vi "Write Conversion Log File.vi"(8 "error in (no error)":errorcluster, 10 "Additional Notes?":string, 11 "Conversion.lvclass":refnum<class "Conversion.lvclass">) -> (0 "error out":errorcluster, 2 "Log File Path":path, 3 "Conversion.lvclass out":refnum<class "Conversion.lvclass">)   [LabVIEW 2016, in "Conversion.lvclass"]
uses:
  Conversion.lvclass
  Conversion.lvclass/Conversion.ctl
  <userlib>/_OpenG.lib/array/array.llb/Remove Duplicates from 1D Array (Path)__ogtk.vi
  <userlib>/_OpenG.lib/file/file.llb/Strip Path - Arrays__ogtk.vi
panel:
  in  "OK":bool
  out "resulting string":string
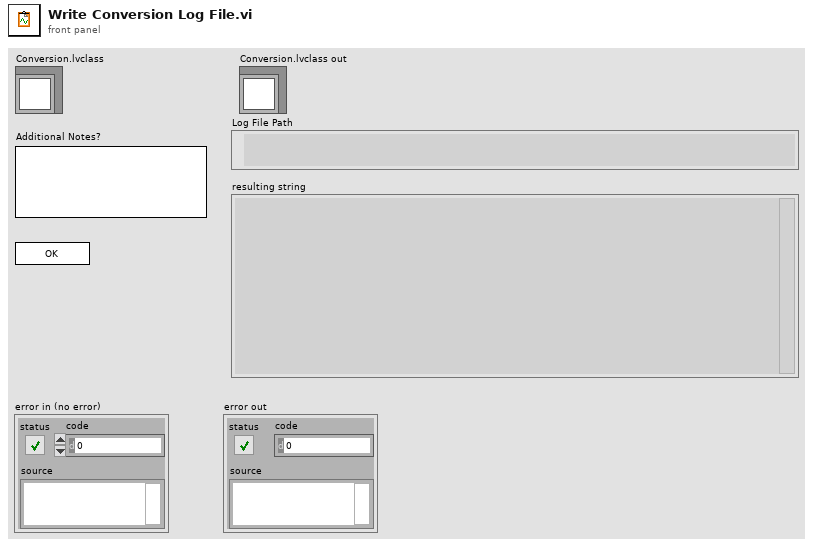
[diagram p1: front panel]
types:
  T1 = enum32{"Invalid", "Standard", "Closed", "Hidden", "Minimized", "Maximized"}
  T2 = enum32{"invalid app kind", "Development System", "Run Time System", "Student Edition", "Embedded LabVIEW", "Evaluation", "Custom"}
  T3 = cluster{"Core":cluster{"Current VI Reference":refnum<vi>, "Close Panel on Exit?":bool}, "Conversion.lvclass":refnum<class "Conversion.lvclass">, "Data.lvclass":refnum<class "Data.lvclass">, "Conversion Start time":timestamp, "Conversion End time":timestamp, "Original":path[], "Converted":path[], "Failed Conversions":path[], "Metadata":cluster{"Instrument":string, "Device":string, "Sample":string, "Experiment":string}, "Log":cluster{"Start Time":string, "End Time":string, "string":string}}
  T4 = cluster{"Instrument":string, "Device":string, "Sample":string, "Experiment":string}
  T5 = cluster{"Start Time":string, "End Time":string, "string":string}
  T6 = cluster{"Current VI Reference":refnum<vi>, "Close Panel on Exit?":bool}
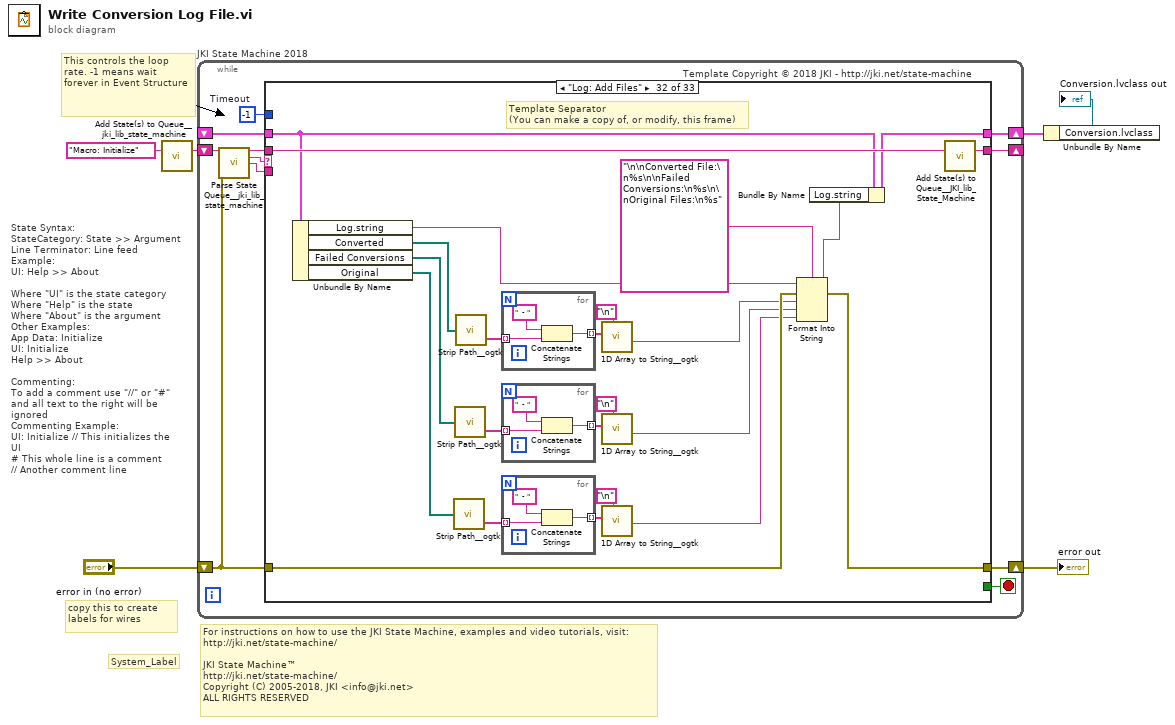
[diagram p0: block diagram]
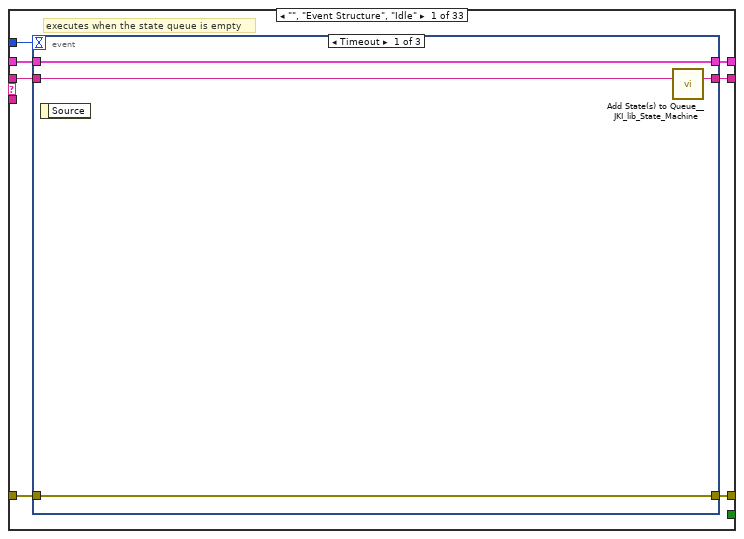
[diagram p2: hidden frame]
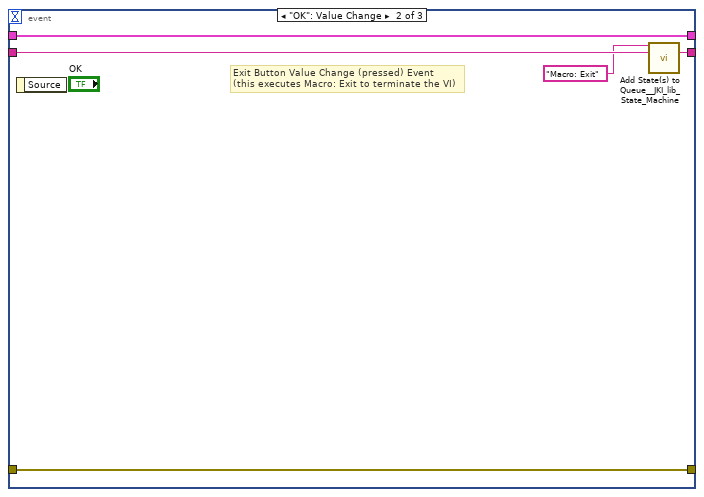
[diagram p3: hidden frame]
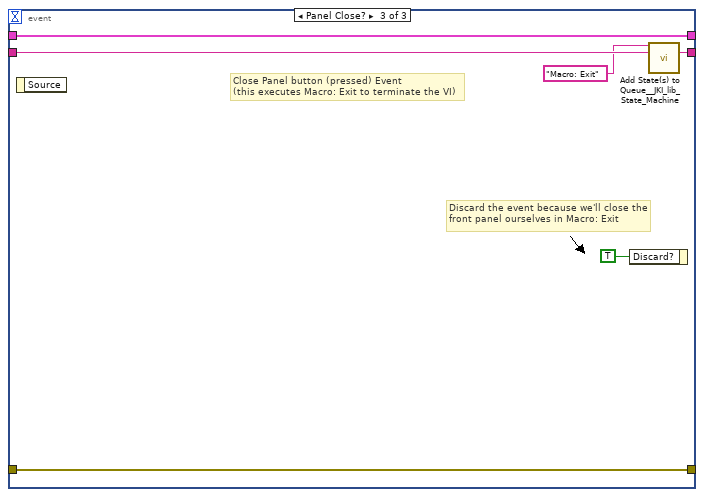
[diagram p4: hidden frame]
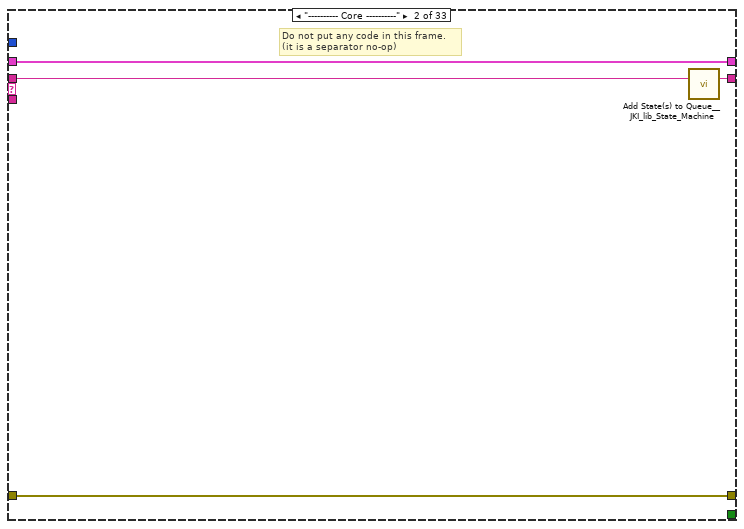
[diagram p5: hidden frame]
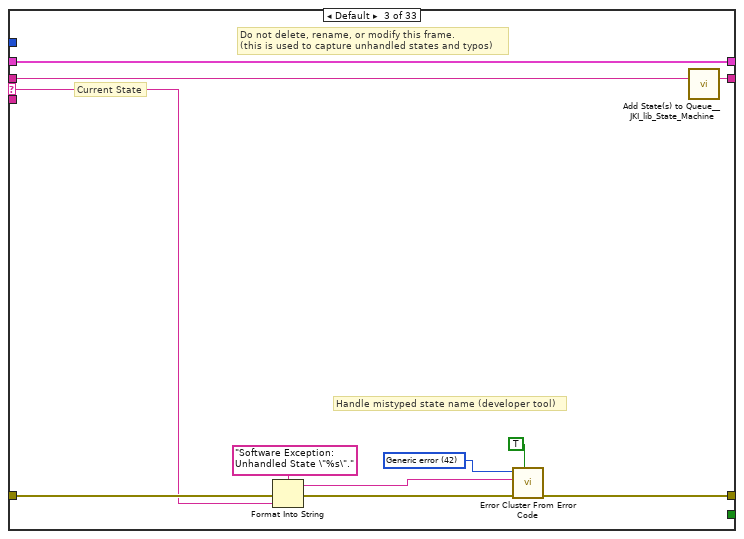
[diagram p6: hidden frame]
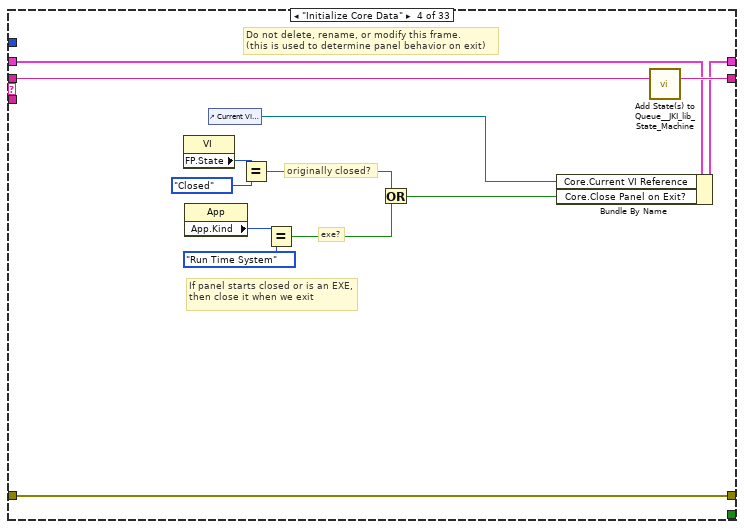
[diagram p7: hidden frame]
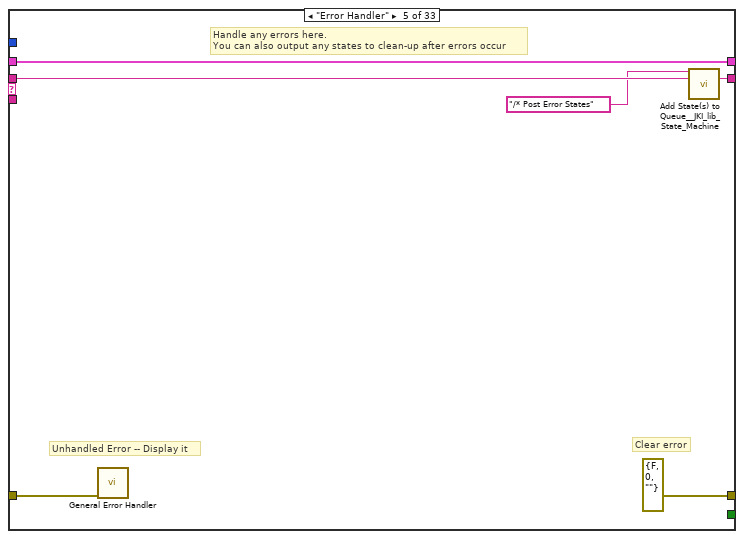
[diagram p8: hidden frame]
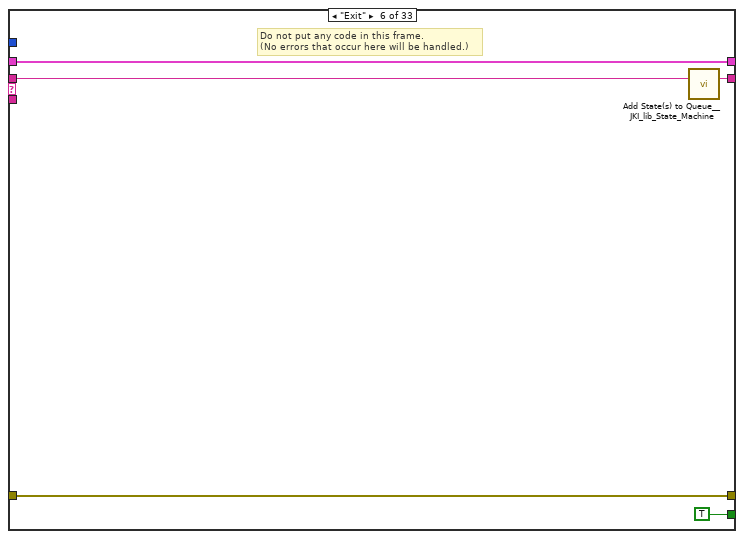
[diagram p9: hidden frame]
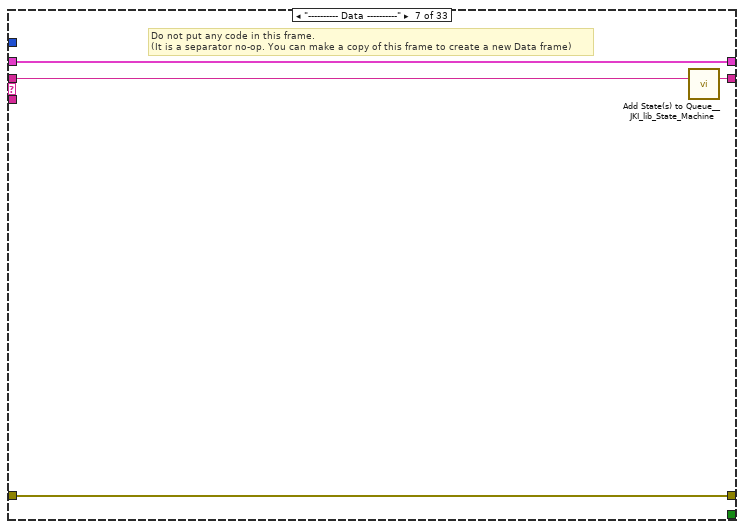
[diagram p10: hidden frame]
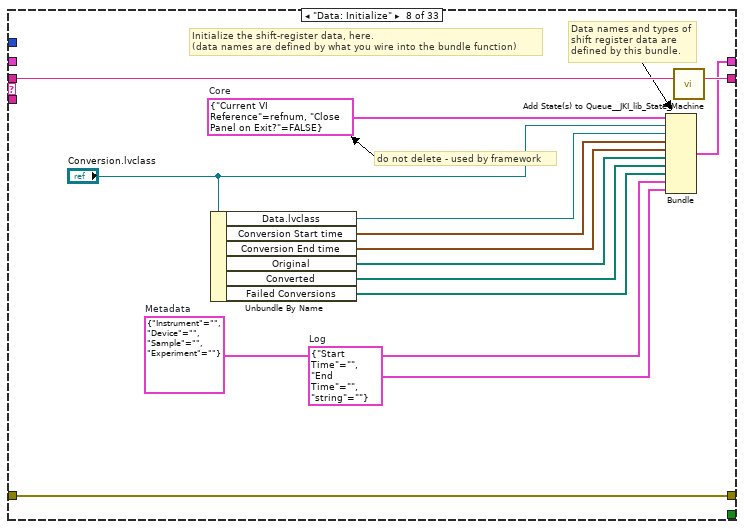
[diagram p11: hidden frame]
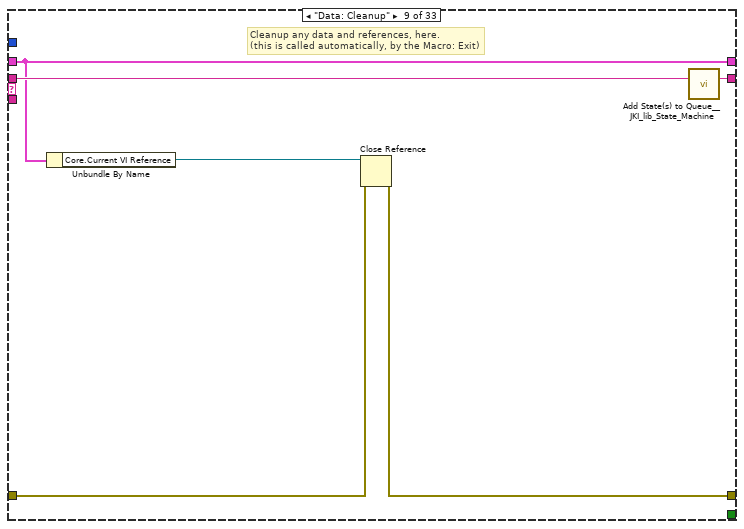
[diagram p12: hidden frame]
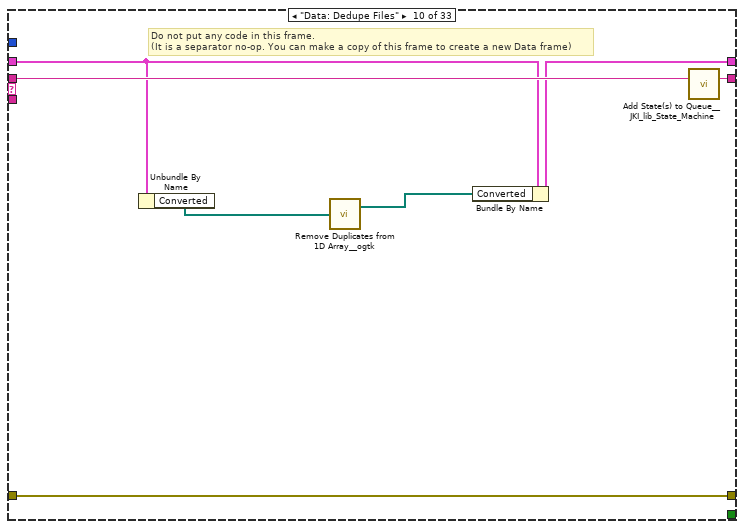
[diagram p13: hidden frame]
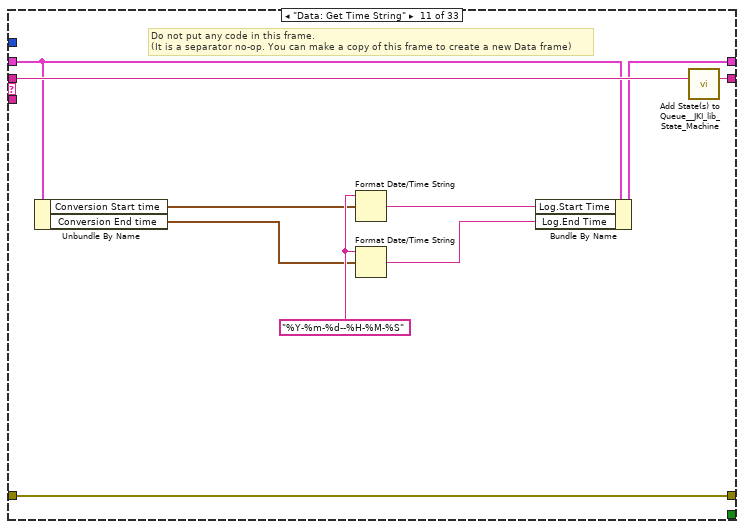
[diagram p14: hidden frame]
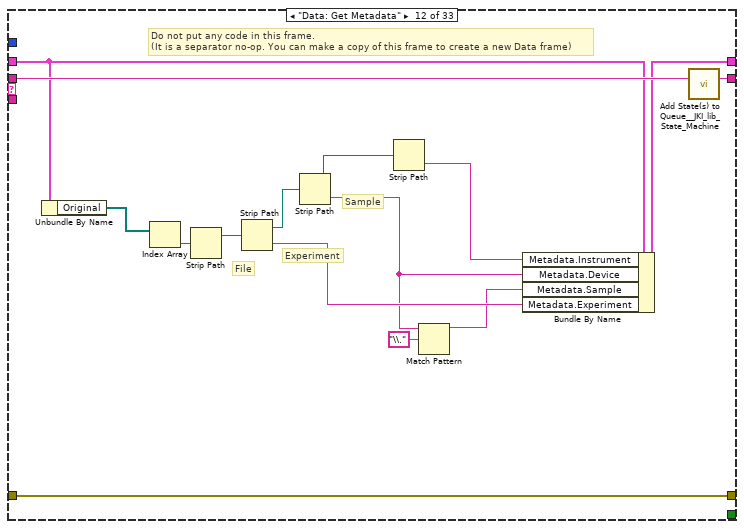
[diagram p15: hidden frame]
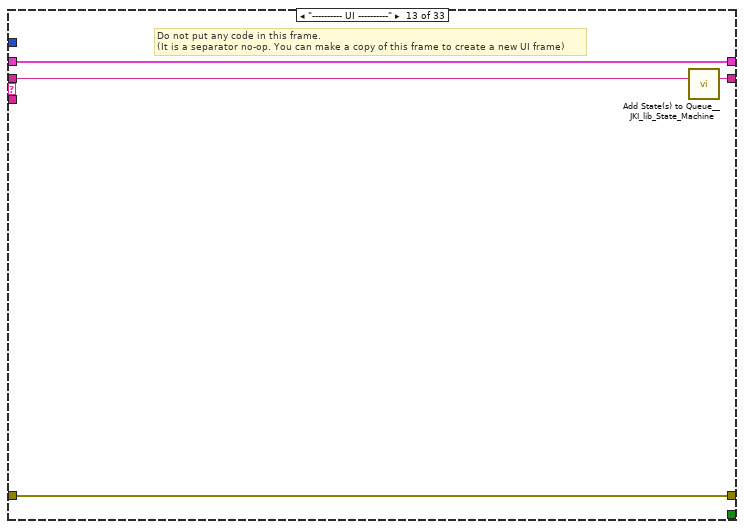
[diagram p16: hidden frame]
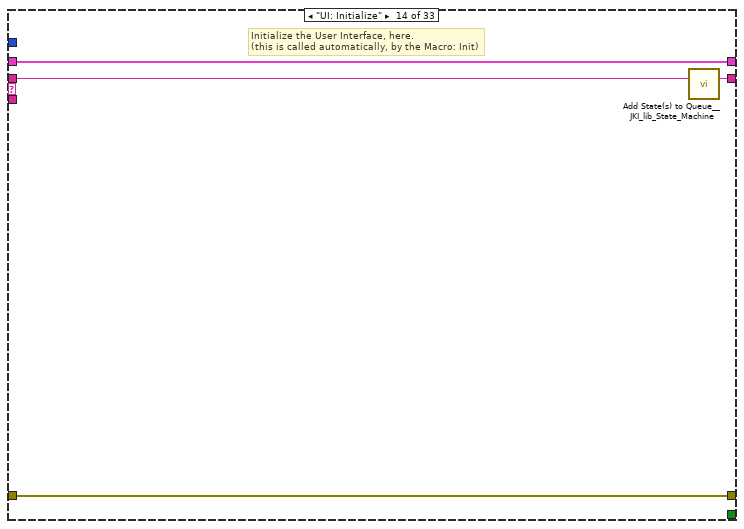
[diagram p17: hidden frame]
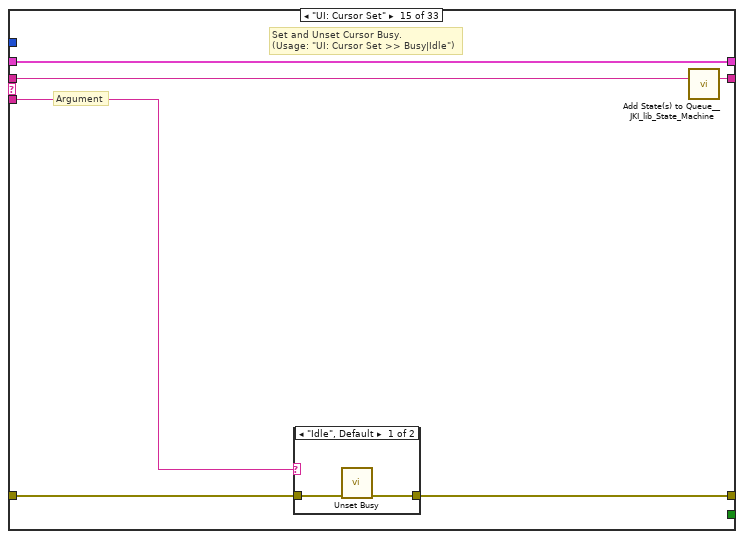
[diagram p18: hidden frame]
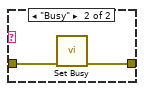
[diagram p19: hidden frame]
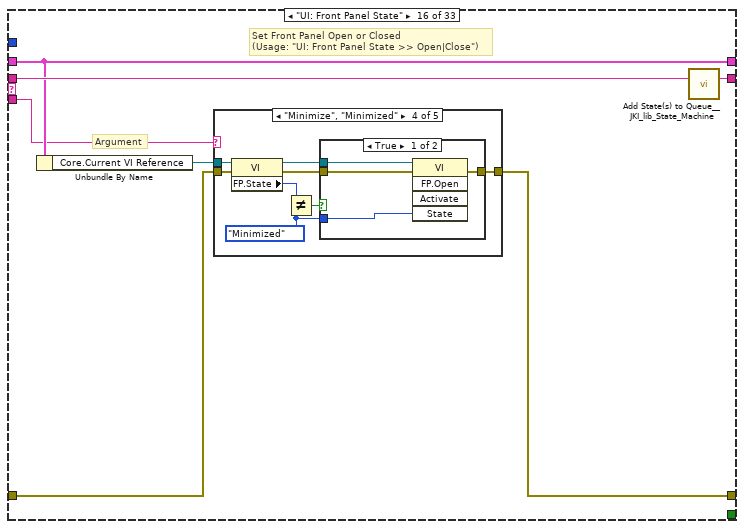
[diagram p20: hidden frame]
diagram:
  # "For instructions on how to use the JKI State Machine, examples and video tutorials, visit:\nhttp://jki.net/state-machine/\n\nJKI State Machine™\nhttp://jki.net/state-machine/\nCopyright (C) 2005-2018, JKI <info@jki.net>\nALL RIGHTS RESERVED"
  # "State Syntax:\nStateCategory: State >> Argument\nLine Terminator: Line feed\nExample:\nUI: Help >> About\n\nWhere \"UI\" is the state category\nWhere \"Help\" is the state\nWhere \"About\" is the argument\nOther Examples:\nApp Data: Initialize\nUI: Initialize\nHelp >> About\n\nCommenting:\nTo add a comment use \"//\" or \"#\" and all text to the right will be ignored\nCommenting Example:\nUI: Initialize // This initializes the UI\n# This whole line is a comment\n// Another comment line"
  # "copy this to create labels for wires"
  # "This controls the loop rate. -1 means wait forever in Event Structure"
  # "System_Label"
  n1 = call <vilib>:"Add State(s) to Queue__jki_lib_state_machine.vi"("State(s) in (\"\")"="Macro: Initialize") -> ("States Out"=w6:string)  [unwired: 14 in]
  n2 = while "JKI State Machine 2018" {
    shift-right: [w10] -> w2
    shift-left: _ -> [w9]
    shift-right: [w13] -> w4
    shift-left: "error in (no error)" -> [w7]
    shift-right: [w12] -> _
    shift-left: w6 -> [w14]
    stop <- w11 stop-if-true
    w8 = -1  # Timeout
    # "Template Copyright © 2018 JKI - http://jki.net/state-machine"
    n3 = call <vilib>:"Parse State Queue__jki_lib_state_machine.vi"("State Queue"=w14, "Error In (no error)"=w7) -> ("Remaining States"=w16:string, "Current State"=w17:string, "Arguments"=w15:string)  [unwired: 11 in]
    n4 = case shown="\"Log: Add Files\"" w17 {
      selector: w17 -> [_ _ w44 _ _ _ _ _ _ _ _ _ _ _ _ _ _ _ _ _ _ _ _ _ _ _ _ _ _ _ _ _ _]
      tunnel: w16 -> [w24 w43 w48 w67 w73 w78 w82 w96 w102 w109 w119 w134 w138 w142 w148 w159 w228 w233 w238 w248 w258 w262 w268 w278 w288 w312 w324 w335 w359 w394 w412 w447 w473]
      tunnel: w15 -> [_ _ _ _ _ _ _ _ _ _ _ _ _ _ w143 w153 _ _ _ _ _ _ _ _ _ _ _ _ _ _ _ _ _]
      tunnel: w9 -> [w22 w40 w46 w60 w70 w76 w79 _ w97 w106 w115 w126 w135 w140 w146 w155 w225 w230 w235 w245 w256 w259 w265 w276 w286 w310 w322 w333 w357 w392 w410 w445 w471]
      tunnel: [w21 w41 w50 w64 errorcluster {"status"=FALSE, "code"=0, "source"=""} ("error out") w75 w80 w93 w98 w107 w117 w132 w136 w139 w144 w156 w226 w231 w236 w246 w250 w260 w266 w271 w280 w301 w316 w327 w354 w387 w401 w440 w467] -> w13
      tunnel: w7 -> [w20 w41 w49 w64 w69 w75 w80 w93 w99 w107 w117 w132 w136 w139 w145 w157 w226 w231 w236 w246 w251 w260 w266 w272 w281 w300 w317 w328 w351 w376 w406 w441 w462]
      tunnel: [w23 w42 w47 w66 w72 w77 w81 w95 w101 w108 w118 w133 w137 w141 w147 w158 w227 w232 w237 w247 w257 w261 w267 w277 w287 w311 w323 w334 w358 w393 w411 w446 w472] -> w12
      tunnel: [_ _ _ _ _ TRUE _ _ _ _ _ _ _ _ _ _ _ _ _ _ _ _ _ _ _ _ _ _ _ _ _ _ _] -> w11
      tunnel: [w19 w40 w46 w65 w70 w76 w79 w94 w97 w104 w112 w125 w135 w140 w146 w155 w225 w230 w235 w245 w255 w259 w264 w275 w285 w309 w321 w332 w356 w391 w409 w444 w471] -> w10
      tunnel: w8 -> [w18 _ _ _ _ _ _ _ _ _ _ _ _ _ _ _ _ _ _ _ _ _ _ _ _ _ _ _ _ _ _ _ _]
      frame "", "Event Structure", "Idle" {
        # "executes when the state queue is empty"
        n5 = event shown="[0] Timeout" {
          selector: _ -> [_ _ _]
          dyn-events: _ -> [_ _ _]
          timeout: w18 -> [_ _ _]
          tunnel: w24 -> [w28 w33 w39]
          tunnel: [w27 w32 w38] -> w23
          tunnel: w22 -> [w25 w30 w36]
          tunnel: [w26 w31 w37] -> w21
          tunnel: w20 -> [w26 w31 w37]
          tunnel: [w25 w30 w36] -> w19
          event Timeout {
            n6 = event-data() -> ()  [unwired: 1 in, 1 out]
            n7 = call <vilib>:"Add State(s) to Queue__JKI_lib_State_Machine.vi"("State(s) in (\"\")"=w28) -> ("States Out"=w27:string)  [unwired: 14 in]
          }
          event "OK": Value Change {
            # "Exit Button Value Change (pressed) Event\n(this executes Macro: Exit to terminate the VI)"
            n8 = event-data() -> ()  [unwired: 1 in, 1 out]
            n9 = call <vilib>:"Add State(s) to Queue__JKI_lib_State_Machine.vi"("State(s) in Front (\"\")"="Macro: Exit", "State(s) in (\"\")"=w33) -> ("States Out"=w32:string)  [unwired: 13 in]
          }
          event Panel Close? {
            # "Discard the event because we'll close the front panel ourselves in Macro: Exit"
            # "Close Panel button (pressed) Event\n(this executes Macro: Exit to terminate the VI)"
            n10 = event-data() -> ()  [unwired: 1 in, 1 out]
            n11 = event-data("Discard?"=TRUE) -> ()  [unwired: 1 in, 1 out]
            n12 = call <vilib>:"Add State(s) to Queue__JKI_lib_State_Machine.vi"("State(s) in Front (\"\")"="Macro: Exit", "State(s) in (\"\")"=w39) -> ("States Out"=w38:string)  [unwired: 13 in]
          }
        }
      }
      frame "---------- Core ----------" {
        # "Do not put any code in this frame.\n(it is a separator no-op)"
        n13 = call <vilib>:"Add State(s) to Queue__JKI_lib_State_Machine.vi"("State(s) in (\"\")"=w43) -> ("States Out"=w42:string)  [unwired: 14 in]
      }
      frame Default {
        w53 = 42 items=["No error", "Argument error", "Memory is full", "Out of zone", "End of file", "File already open", "Generic file I/O error", "File not found", "File permission error", "Disk is full", "Duplicate path", "Too many files open", "System feature not enabled", "Resource file not found", "Cannot add resource", "Resource not found", "Image not found", "Image memory error", "Pen does not exist", "Config type invalid", "Config token not found", "Config parse error", "Config memory error", "Bad external code format", "Bad external code offset", "External code not present", "Null window", "Destroy window error", "Null menu", "Print aborted", "Bad print record", "Print driver error", "Windows error during printing", "Memory error during printing", "Print dialog error", "Generic print error", "Invalid device refnum", "Device not found", "Device parameter error", "Device unit error", "Cannot open device", "Device call aborted", "Generic error", "Cancelled by user", "Object ID too low", "Object ID too high", "Object not in heap", "Unknown heap", "Unknown object (invalid DefProc)", "Unknown object (DefProc not in table)", "Message out of range", "Invalid (null) method", "Unknown message", "Manager call not supported", "Bad address", "Network operation in progress", "Network operation timed out", "Connection is busy", "Network attribute not supported", "Network error", "Address in use", "System out of memory", "Connection aborted", "Connection refused", "Not connected", "Already connected", "Connection closed", "Initialization error (interapplication manager)", "Bad occurrence", "Wait on unbound occurrence handler", "Occurrence queue overflow", "Datalog type conflict", "Unused", "Unrecognized type (interapplication manager)", "Memory corrupt", "Failed to make temporary DLL", "Old CIN version", "Drag socket not found", "Failed to load drop-object", "Failed to register OLE object", "Failed to release OLE object", "Format specifier type mismatch", "Unknown format specifier", "Too few format specifiers", "Too many format specifiers", "Scan failed", "Newer CIN version", "Error converting to variant", "Runtime menu error", "Password tampered", "Variant attribute not found", "Incompatible variant data type", "Event data is not available", "Event Store is not present", "Occurrence is not found", "Event Queue is not created", "Event info is not available", "Refnum passed is NULL", "Error retrieving Class GUID", "Error retrieving CoClass GUID", "Error retrieving TypeLib GUID.", "Bad built application magic bytes.", "Specific driver is different from the specific driver associated with the Logical Name.", "There is no session opened to the class driver.", "Max Error", "MAX - Error with config objects", "MAX - Error loading configuration", "MAX - Group not supported"]
        # "Current State"
        # "Do not delete, rename, or modify this frame.\n(this is used to capture unhandled states and typos)"
        # "Handle mistyped state name (developer tool)"
        n14 = Format Into String(format string="Software Exception: Unhandled State \"%s\"." ("message"), error in=w49, w44) -> (resulting string=w52:string, error out=w51:errorcluster)  [unwired: 1 in]
        n15 = call <vilib>:"Error Cluster From Error Code.vi"("show call chain? (False)"=TRUE, "error in (no error)"=w51, "error message (\"\")"=w52, "error code (0)"=w53) -> ("error out"=w50:errorcluster)  [unwired: 5 in]
        n16 = call <vilib>:"Add State(s) to Queue__JKI_lib_State_Machine.vi"("State(s) in (\"\")"=w48) -> ("States Out"=w47:string)  [unwired: 14 in]
      }
      frame "Initialize Core Data" {
        # "Do not delete, rename, or modify this frame.\n(this is used to determine panel behavior on exit)"
        # "originally closed?"
        # "exe?"
        # "If panel starts closed or is an EXE, then close it when we exit"
        n17 = property class="VI"() -> ("FP.State"=w57:T1)  [unwired: 2 in, 2 out]
        n18 = property class="App"() -> ("App.Kind"=w63:T2)  [unwired: 2 in, 2 out]
        n19 = control-ref of="Current VI Reference"() -> (w58:refnum<vi>)
        n20 = Equal?(x=w57, y=T1."Closed" ("Front Panel Window:State")) -> (x = y?=w55:bool)
        n21 = Equal?(x=w63, y=T2."Run Time System" ("Application:Kind")) -> (x = y?=w61:bool)
        n22 = Or(x=w55, y=w61) -> (x .or. y?=w59:bool)
        n23 = Bundle By Name(cluster=w60, "Core.Current VI Reference"=w58, "Core.Close Panel on Exit?"=w59) -> (w65:T3)
        n24 = call <vilib>:"Add State(s) to Queue__JKI_lib_State_Machine.vi"("State(s) in (\"\")"=w67) -> ("States Out"=w66:string)  [unwired: 14 in]
      }
      frame "Error Handler" {
        # "Unhandled Error -- Display it"
        # "Handle any errors here.\nYou can also output any states to clean-up after errors occur"
        # "Clear error"
        n25 = call <vilib>:"General Error Handler.vi"("error in (no error)"=w69) -> ()  [unwired: 10 in, 5 out]
        n26 = call <vilib>:"Add State(s) to Queue__JKI_lib_State_Machine.vi"("State(s) in Front (\"\")"="/* Post Error States", "State(s) in (\"\")"=w73) -> ("States Out"=w72:string)  [unwired: 13 in]
      }
      frame "Exit" {
        # "Do not put any code in this frame.\n(No errors that occur here will be handled.)"
        n27 = call <vilib>:"Add State(s) to Queue__JKI_lib_State_Machine.vi"("State(s) in (\"\")"=w78) -> ("States Out"=w77:string)  [unwired: 14 in]
      }
      frame "---------- Data ----------" {
        # "Do not put any code in this frame.\n(It is a separator no-op. You can make a copy of this frame to create a new Data frame)"
        n28 = call <vilib>:"Add State(s) to Queue__JKI_lib_State_Machine.vi"("State(s) in (\"\")"=w82) -> ("States Out"=w81:string)  [unwired: 14 in]
      }
      frame "Data: Initialize" {
        w85 = T4 {"Instrument"="", "Device"="", "Sample"="", "Experiment"=""}  # Metadata
        w86 = T5 {"Start Time"="", "End Time"="", "string"=""}  # Log
        w92 = T6 {"Current VI Reference"=refnum, "Close Panel on Exit?"=FALSE}  # Core
        # "do not delete - used by framework"
        # "Data names and types of shift register data are defined by this bundle."
        # "Initialize the shift-register data, here.\n(data names are defined by what you wire into the bundle function)"
        n29 = Unbundle By Name("Conversion.lvclass") -> ("Data.lvclass"=w91:refnum<class "Data.lvclass">, "Conversion Start time"=w90:timestamp, "Conversion End time"=w89:timestamp, "Original"=w87:path[], "Converted"=w84:path[], "Failed Conversions"=w88:path[])
        n30 = Bundle("Core"=w92, "Conversion.lvclass"="Conversion.lvclass", "Data.lvclass"=w91, "Conversion Start time"=w90, "Conversion End time"=w89, "Original"=w87, "Converted"=w84, "Failed Conversions"=w88, "Metadata"=w85, "Log"=w86) -> (w94:T3)  [unwired: 1 in]
        n31 = call <vilib>:"Add State(s) to Queue__JKI_lib_State_Machine.vi"("State(s) in (\"\")"=w96) -> ("States Out"=w95:string)  [unwired: 14 in]
      }
      frame "Data: Cleanup" {
        # "Cleanup any data and references, here.\n(this is called automatically, by the Macro: Exit)"
        n32 = Unbundle By Name(w97) -> ("Core.Current VI Reference"=w100:refnum<vi>)
        n33 = Close Reference(reference=w100, error in (no error)=w99) -> (error out=w98:errorcluster)
        n34 = call <vilib>:"Add State(s) to Queue__JKI_lib_State_Machine.vi"("State(s) in (\"\")"=w102) -> ("States Out"=w101:string)  [unwired: 14 in]
      }
      frame "Data: Dedupe Files" {
        # "Do not put any code in this frame.\n(It is a separator no-op. You can make a copy of this frame to create a new Data frame)"
        n35 = Unbundle By Name(w106) -> ("Converted"=w105:path[])
        n36 = call-poly <userlib>:"Remove Duplicates from 1D Array__ogtk.vi"("Input Array"=w105) -> ("Output Array"=w103:path[])  [unwired: 1 out]
        n37 = Bundle By Name(cluster=w106, "Converted"=w103) -> (w104:T3)
        n38 = call <vilib>:"Add State(s) to Queue__JKI_lib_State_Machine.vi"("State(s) in (\"\")"=w109) -> ("States Out"=w108:string)  [unwired: 14 in]
      }
      frame "Data: Get Time String" {
        w116 = "%Y-%m-%d--%H-%M-%S" ("time format string (%c)")
        # "Do not put any code in this frame.\n(It is a separator no-op. You can make a copy of this frame to create a new Data frame)"
        n39 = Unbundle By Name(w115) -> ("Conversion Start time"=w114:timestamp, "Conversion End time"=w113:timestamp)
        n40 = Format Date/Time String(time format string (%c)=w116, seconds (now)=w114) -> (date/time string=w111:string)  [unwired: 1 in]
        n41 = Format Date/Time String(time format string (%c)=w116, seconds (now)=w113) -> (date/time string=w110:string)  [unwired: 1 in]
        n42 = Bundle By Name(cluster=w115, "Log.Start Time"=w111, "Log.End Time"=w110) -> (w112:T3)
        n43 = call <vilib>:"Add State(s) to Queue__JKI_lib_State_Machine.vi"("State(s) in (\"\")"=w119) -> ("States Out"=w118:string)  [unwired: 14 in]
      }
      frame "Data: Get Metadata" {
        # "Sample"
        # "Experiment"
        # "File"
        # "Do not put any code in this frame.\n(It is a separator no-op. You can make a copy of this frame to create a new Data frame)"
        n44 = Unbundle By Name(w126) -> ("Original"=w127:path[])
        n45 = Index Array(array=w127) -> (element=w130:path)  [unwired: 1 in]
        n46 = Strip Path(path=w130) -> (stripped path=w129:path)  [unwired: 1 out]
        n47 = Strip Path(path=w129) -> (stripped path=w131:path, name=w123:string)
        n48 = Strip Path(path=w131) -> (stripped path=w128:path, name=w122:string)
        n49 = Strip Path(path=w128) -> (name=w124:string)  [unwired: 1 out]
        n50 = Match Pattern(string=w122, regular expression="\\.") -> (before substring=w120:string)  [unwired: 1 in, 3 out]
        n51 = Bundle By Name(cluster=w126, "Metadata.Instrument"=w124, "Metadata.Device"=w122, "Metadata.Sample"=w120, "Metadata.Experiment"=w123) -> (w125:T3)
        n52 = call <vilib>:"Add State(s) to Queue__JKI_lib_State_Machine.vi"("State(s) in (\"\")"=w134) -> ("States Out"=w133:string)  [unwired: 14 in]
      }
      frame "---------- UI ----------" {
        # "Do not put any code in this frame.\n(It is a separator no-op. You can make a copy of this frame to create a new UI frame)"
        n53 = call <vilib>:"Add State(s) to Queue__JKI_lib_State_Machine.vi"("State(s) in (\"\")"=w138) -> ("States Out"=w137:string)  [unwired: 14 in]
      }
      frame "UI: Initialize" {
        # "Initialize the User Interface, here.\n(this is called automatically, by the Macro: Init)"
        n54 = call <vilib>:"Add State(s) to Queue__JKI_lib_State_Machine.vi"("State(s) in (\"\")"=w142) -> ("States Out"=w141:string)  [unwired: 14 in]
      }
      frame "UI: Cursor Set" {
        # "Argument"
        # "Set and Unset Cursor Busy.\n(Usage: \"UI: Cursor Set >> Busy|Idle\")"
        n55 = case shown="\"Idle\", Default" w143 {
          tunnel: w145 -> [w150 w152]
          tunnel: [w149 w151] -> w144
          frame "Idle", Default {
            n56 = call <vilib>:"Unset Busy.vi"("error in (no error)"=w150) -> ("error out"=w149:errorcluster)  [unwired: 10 in]
          }
          frame "Busy" {
            n57 = call <vilib>:"Set Busy.vi"("error in (no error)"=w152) -> ("error out"=w151:errorcluster)  [unwired: 9 in, 1 out]
          }
        }
        n58 = call <vilib>:"Add State(s) to Queue__JKI_lib_State_Machine.vi"("State(s) in (\"\")"=w148) -> ("States Out"=w147:string)  [unwired: 14 in]
      }
      frame "UI: Front Panel State" {
        # "Argument"
        # "Set Front Panel Open or Closed\n(Usage: \"UI: Front Panel State >> Open|Close\")"
        n59 = Unbundle By Name(w155) -> ("Core.Current VI Reference"=w154:refnum<vi>)
        n60 = case shown="\"Minimize\", \"Minimized\"" w153 {
          tunnel: w157 -> [w165 w180 w191 w204 w217]
          tunnel: [w167 w181 w193 w206 w219] -> w156
          tunnel: w154 -> [w166 w178 w192 w205 w218]
          frame "Open", "Standard", Default {
            w160 = T1."Standard" ("State")
            n61 = property class="VI"(reference=w166, error in=w165) -> (reference out=w163:refnum<vi>, error out=w164:errorcluster, "FP.State"=w162:T1)
            n62 = Not Equal?(x=w162, y=w160) -> (x != y?=w161:bool)
            n63 = case shown="True" w161 {
              tunnel: [w171 w173] -> w167
              tunnel: w164 -> [w170 w173]
              tunnel: w163 -> [w169 _]
              tunnel: w160 -> [w168 _]
              frame True {
                n64 = invoke class="VI" method="FP.Open"(reference=w169, error in=w170, "Activate"=TRUE, "State"=w168) -> (error out=w171:errorcluster)  [unwired: 1 in, 4 out]
              }
              frame False {
              }
            }
          }
          frame "Close", "Closed" {
            n65 = property class="VI"(reference=w178, error in=w180) -> (reference out=w177:refnum<vi>, error out=w179:errorcluster, "FP.State"=w175:T1)
            n66 = Not Equal?(x=w175, y=T1."Closed" ("Front Panel Window:State")) -> (x != y?=w174:bool)
            n67 = case shown="True" w174 {
              tunnel: [w182 w185] -> w181
              tunnel: w179 -> [w182 w184]
              tunnel: w177 -> [_ w183]
              frame False {
              }
              frame True {
                n68 = invoke class="VI" method="FP.Close"(reference=w183, error in=w184) -> (error out=w185:errorcluster)  [unwired: 1 in, 2 out]
              }
            }
          }
          frame "Hidden", "Hide" {
            w186 = T1."Hidden" ("State")
            n69 = property class="VI"(reference=w192, error in=w191) -> (reference out=w189:refnum<vi>, error out=w190:errorcluster, "FP.State"=w188:T1)
            n70 = Not Equal?(x=w188, y=w186) -> (x != y?=w187:bool)
            n71 = case shown="True" w187 {
              tunnel: [w197 w198] -> w193
              tunnel: w190 -> [w196 w198]
              tunnel: w189 -> [w195 _]
              tunnel: w186 -> [w194 _]
              frame True {
                n72 = invoke class="VI" method="FP.Open"(reference=w195, error in=w196, "State"=w194) -> (error out=w197:errorcluster)  [unwired: 2 in, 4 out]
              }
              frame False {
              }
            }
          }
          frame "Minimize", "Minimized" {
            w199 = T1."Minimized" ("State")
            n73 = property class="VI"(reference=w205, error in=w204) -> (reference out=w202:refnum<vi>, error out=w203:errorcluster, "FP.State"=w201:T1)
            n74 = Not Equal?(x=w201, y=w199) -> (x != y?=w200:bool)
            n75 = case shown="True" w200 {
              tunnel: [w210 w211] -> w206
              tunnel: w203 -> [w209 w211]
              tunnel: w202 -> [w208 _]
              tunnel: w199 -> [w207 _]
              frame True {
                n76 = invoke class="VI" method="FP.Open"(reference=w208, error in=w209, "State"=w207) -> (error out=w210:errorcluster)  [unwired: 2 in, 4 out]
              }
              frame False {
              }
            }
          }
          frame "Maximize", "Maximized" {
            w212 = T1."Maximized" ("State")
            n77 = property class="VI"(reference=w218, error in=w217) -> (reference out=w215:refnum<vi>, error out=w216:errorcluster, "FP.State"=w214:T1)
            n78 = Not Equal?(x=w214, y=w212) -> (x != y?=w213:bool)
            n79 = case shown="True" w213 {
              tunnel: [w223 w224] -> w219
              tunnel: w216 -> [w222 w224]
              tunnel: w215 -> [w221 _]
              tunnel: w212 -> [w220 _]
              frame True {
                n80 = invoke class="VI" method="FP.Open"(reference=w221, error in=w222, "State"=w220) -> (error out=w223:errorcluster)  [unwired: 2 in, 4 out]
              }
              frame False {
              }
            }
          }
        }
        n81 = call <vilib>:"Add State(s) to Queue__JKI_lib_State_Machine.vi"("State(s) in (\"\")"=w159) -> ("States Out"=w158:string)  [unwired: 14 in]
      }
      frame "---------- Macro ----------" {
        # "Do not put any code in this frame.\n(It is a separator no-op. You can make a copy of this frame to create a new Macro frame)"
        n82 = call <vilib>:"Add State(s) to Queue__JKI_lib_State_Machine.vi"("State(s) in (\"\")"=w228) -> ("States Out"=w227:string)  [unwired: 14 in]
      }
      frame "Macro: Initialize" {
        w229 = "Data: Initialize\nInitialize Core Data\nUI: Initialize\nUI: Front Panel State >> Open\nMacro: Log\nMacro: Exit"  # Data: Initialize Initialize Core Data UI: Initialize UI: Front Panel State >> Open Macro: Log Macro: Exit
        # "Initialization Macro\n(This is called once, when the VI starts)"
        n83 = call <vilib>:"Add State(s) to Queue__JKI_lib_State_Machine.vi"("State(s) in Front (\"\")"=w229, "State(s) in (\"\")"=w233) -> ("States Out"=w232:string)  [unwired: 13 in]
      }
      frame "Macro: Log" {
        # "Initialization Macro\n(This is called once, when the VI starts)"
        n84 = call <vilib>:"Add State(s) to Queue__JKI_lib_State_Machine.vi"("State(s) in Front (\"\")"="Log: Temp\nData: Dedupe Files\nData: Get Time String\nData: Get Metadata\nLog: Initialize\nLog: Add Start Time\nLog: Add End Time\nLog: Add Number and Elapsed Time\nLog: Add Original Folder Name\nLog: Add Converted Folder Name\nLog: Add Number of Files\nLog: Add File Sizes\nLog: Add Notes\nLog: Add Files\nLog: Write File", "State(s) in (\"\")"=w238) -> ("States Out"=w237:string)  [unwired: 13 in]
      }
      frame "Macro: Exit" {
        # "Exit Macro\n(This is called once, when the VI exits)"
        n85 = Unbundle By Name(w245) -> ("Core.Close Panel on Exit?"=w244:bool)
        n86 = Select(t="UI: Front Panel State >> Close", s=w244, f="") -> (s? t:f=w241:string)
        n87 = call <vilib>:"Add State(s) to Queue__JKI_lib_State_Machine.vi"("State(s) in (\"\")"=w241, "State(s) at Back (\"\")"="Data: Cleanup\nExit") -> ("States Out"=w239:string)  [unwired: 13 in]
        n88 = call <vilib>:"Add State(s) to Queue__JKI_lib_State_Machine.vi"("State(s) in Front (\"\")"=w239, "State(s) in (\"\")"=w248) -> ("States Out"=w247:string)  [unwired: 13 in]
      }
      frame "---------- Log ----------" {
        # "Template Separator\n(You can make a copy of, or modify, this frame)"
        n89 = Unbundle By Name(w256) -> ("Log.string"=w253:string)
        n90 = Format Into String(format string="\n%s", initial string=w253, error in=w251, "" ("input 1")) -> (resulting string=w252:string, error out=w250:errorcluster)
        n91 = Bundle By Name(cluster=w256, "Log.string"=w252) -> (w255:T3)
        n92 = call <vilib>:"Add State(s) to Queue__JKI_lib_State_Machine.vi"("State(s) in (\"\")"=w258) -> ("States Out"=w257:string)  [unwired: 14 in]
      }
      frame "Log: Temp" {
        # "Your code here.\n(You can make a copy of, or modify, this frame)"
        n93 = call <vilib>:"Add State(s) to Queue__JKI_lib_State_Machine.vi"("State(s) in (\"\")"=w262) -> ("States Out"=w261:string)  [unwired: 14 in]
      }
      frame "Log: Initialize" {
        w263 = "Data File Conversion Summary"  # new
        # "Template Separator\n(You can make a copy of, or modify, this frame)"
        n94 = Bundle By Name(cluster=w265, "Log.string"=w263) -> (w264:T3)
        n95 = call <vilib>:"Add State(s) to Queue__JKI_lib_State_Machine.vi"("State(s) in (\"\")"=w268) -> ("States Out"=w267:string)  [unwired: 14 in]
      }
      frame "Log: Add Start Time" {
        # "Template Separator\n(You can make a copy of, or modify, this frame)"
        n96 = Unbundle By Name(w276) -> ("Log.string"=w270:string, "Log.Start Time"=w273:string)
        n97 = Format Into String(format string="\n- Start Time: %s", initial string=w270, error in=w272, w273) -> (resulting string=w269:string, error out=w271:errorcluster)
        n98 = Bundle By Name(cluster=w276, "Log.string"=w269) -> (w275:T3)
        n99 = call <vilib>:"Add State(s) to Queue__JKI_lib_State_Machine.vi"("State(s) in (\"\")"=w278) -> ("States Out"=w277:string)  [unwired: 14 in]
      }
      frame "Log: Add End Time" {
        # "Template Separator\n(You can make a copy of, or modify, this frame)"
        n100 = Unbundle By Name(w286) -> ("Log.string"=w283:string, "Log.End Time"=w282:string)
        n101 = Format Into String(format string="\n- End Time: %s", initial string=w283, error in=w281, w282) -> (resulting string=w279:string, error out=w280:errorcluster)
        n102 = Bundle By Name(cluster=w286, "Log.string"=w279) -> (w285:T3)
        n103 = call <vilib>:"Add State(s) to Queue__JKI_lib_State_Machine.vi"("State(s) in (\"\")"=w288) -> ("States Out"=w287:string)  [unwired: 14 in]
      }
      frame "Log: Add Number and Elapsed Time" {
        # "Template Separator\n(You can make a copy of, or modify, this frame)"
        n104 = Unbundle By Name(w310) -> ("Log.string"=w308:string, "Original"=w307:path[], "Conversion End time"=w298:timestamp, "Conversion Start time"=w299:timestamp)
        n105 = Subtract(x=w298, y=w299) -> (x-y=w304:dbl)
        n106 = Array Size(array=w307) -> (size(s)=w289:i32)
        n107 = Equal?(x=w289, y=1) -> (x = y?=w296:bool)
        n108 = Divide(x=w304, y=w289) -> (x/y=w305:dbl)
        n109 = Select(t="- %d File " ("format string"), s=w296, f="- %d Files " ("format string")) -> (s? t:f=w291:string)
        n110 = Multiply(x=w305, y=1000.0) -> (x*y=w302:dbl)
        n111 = Concatenate Strings("\n", w291, "converted in %d seconds (%d ms/file)" ("format string")) -> (w290:string)
        n112 = Format Into String(format string=w290, initial string=w308, error in=w300, w289, w304, w302) -> (resulting string=w303:string, error out=w301:errorcluster)
        n113 = Bundle By Name(cluster=w310, "Log.string"=w303) -> (w309:T3)
        n114 = call <vilib>:"Add State(s) to Queue__JKI_lib_State_Machine.vi"("State(s) in (\"\")"=w312) -> ("States Out"=w311:string)  [unwired: 14 in]
      }
      frame "Log: Add Original Folder Name" {
        # "Template Separator\n(You can make a copy of, or modify, this frame)"
        n115 = Unbundle By Name(w322) -> ("Log.string"=w319:string, "Original"=w314:path[])
        n116 = Index Array(array=w314) -> (element=w315:path)  [unwired: 1 in]
        n117 = Strip Path(path=w315) -> (stripped path=w313:path)  [unwired: 1 out]
        n118 = Format Into String(format string="\n- Original Folder: %s", initial string=w319, error in=w317, w313) -> (resulting string=w318:string, error out=w316:errorcluster)
        n119 = Bundle By Name(cluster=w322, "Log.string"=w318) -> (w321:T3)
        n120 = call <vilib>:"Add State(s) to Queue__JKI_lib_State_Machine.vi"("State(s) in (\"\")"=w324) -> ("States Out"=w323:string)  [unwired: 14 in]
      }
      frame "Log: Add Converted Folder Name" {
        # "Template Separator\n(You can make a copy of, or modify, this frame)"
        n121 = Unbundle By Name(w333) -> ("Log.string"=w330:string, "Converted"=w326:path[])
        n122 = Index Array(array=w326) -> (element=w325:path)  [unwired: 1 in]
        n123 = Format Into String(format string="\n- Converted File: %s", initial string=w330, error in=w328, w325) -> (resulting string=w329:string, error out=w327:errorcluster)
        n124 = Bundle By Name(cluster=w333, "Log.string"=w329) -> (w332:T3)
        n125 = call <vilib>:"Add State(s) to Queue__JKI_lib_State_Machine.vi"("State(s) in (\"\")"=w335) -> ("States Out"=w334:string)  [unwired: 14 in]
      }
      frame "Log: Add Number of Files" {
        # "Template Separator\n(You can make a copy of, or modify, this frame)"
        n126 = Unbundle By Name(w357) -> ("Log.string"=w355:string, "Original"=w353:path[], "Converted"=w352:path[])
        n127 = Array Size(array=w353) -> (size(s)=w347:i32)
        n128 = Array Size(array=w352) -> (size(s)=w339:i32)
        n129 = Equal?(x=w347, y=1) -> (x = y?=w345:bool)
        n130 = Equal?(x=w339, y=1) -> (x = y?=w341:bool)
        n131 = Select(t="- %d ITX file " ("format string"), s=w345, f="- %d ITX files " ("format string")) -> (s? t:f=w344:string)
        n132 = Select(t="converted to %d TDMS file" ("format string"), s=w341, f="converted to %d TDMS files" ("format string")) -> (s? t:f=w336:string)
        n133 = Concatenate Strings("\n", w344, w336) -> (w348:string)
        n134 = Format Into String(format string=w348, initial string=w355, error in=w351, w347, w339) -> (resulting string=w350:string, error out=w354:errorcluster)
        n135 = Bundle By Name(cluster=w357, "Log.string"=w350) -> (w356:T3)
        n136 = call <vilib>:"Add State(s) to Queue__JKI_lib_State_Machine.vi"("State(s) in (\"\")"=w359) -> ("States Out"=w358:string)  [unwired: 14 in]
      }
      frame "Log: Add File Sizes" {
        w360 = "MB"
        w361 = "KB"
        w368 = i64 1048576 ("y")
        w371 = i64 1048576 ("y")
        # "Template Separator\n(You can make a copy of, or modify, this frame)"
        n137 = Unbundle By Name(w392) -> ("Log.string"=w389:string, "Original"=w385:path[], "Converted"=w382:path[])
        n138 = for {
          tunnel: [w398] -> w386 mode=indexing
          tunnel: w385 -> [w397] mode=indexing
          n139 = File/Directory Info(path=w397) -> (size=w398:i64)  [unwired: 1 in, 6 out]
        }
        n140 = for {
          tunnel: [w396] -> w383 mode=indexing
          tunnel: w382 -> [w395] mode=indexing
          n141 = File/Directory Info(path=w395) -> (size=w396:i64)  [unwired: 1 in, 6 out]
        }
        n142 = Add Array Elements(numeric array=w386) -> (sum=w375:i64)
        n143 = Add Array Elements(numeric array=w383) -> (sum=w372:i64)
        n144 = Less Or Equal?(x=w372, y=w368) -> (x <= y?=w364:bool)
        n145 = Less Or Equal?(x=w375, y=w371) -> (x <= y?=w365:bool)
        n146 = Select(t=i64 1024, s=w365, f=w371) -> (s? t:f=w373:i64)
        n147 = Select(t=i64 1024, s=w364, f=w368) -> (s? t:f=w370:i64)
        n148 = Select(t=w361, s=w365, f=w360) -> (s? t:f=w363:string)
        n149 = Select(t=w361, s=w364, f=w360) -> (s? t:f=w362:string)
        n150 = Divide(x=w375, y=w373) -> (x/y=w377:dbl)
        n151 = Divide(x=w372, y=w370) -> (x/y=w378:dbl)
        n152 = To Long Integer(number=w377) -> (32bit integer=w384:i32)
        n153 = To Long Integer(number=w378) -> (32bit integer=w366:i32)
        n154 = Divide(x=w378, y=w377) -> (x/y=w379:dbl)
        n155 = Multiply(x=w379, y=100.0) -> (x*y=w381:dbl)
        n156 = To Long Integer(number=w381) -> (32bit integer=w367:i32)
        n157 = Format Into String(format string="\n- Original Folder Size: %d %s\n- Converted Folder Size: %d %s\n- The Converted File is %d\\% of the size of the Original", initial string=w389, error in=w376, w384, w363, w366, w362, w367) -> (resulting string=w388:string, error out=w387:errorcluster)
        n158 = Bundle By Name(cluster=w392, "Log.string"=w388) -> (w391:T3)
        n159 = call <vilib>:"Add State(s) to Queue__JKI_lib_State_Machine.vi"("State(s) in (\"\")"=w394) -> ("States Out"=w393:string)  [unwired: 14 in]
      }
      frame "Log: Add Notes" {
        # "Template Separator\n(You can make a copy of, or modify, this frame)"
        n160 = call <userlib>:"Multi-line String to Array__ogtk.vi"("string"="Additional Notes?") -> ("lines"=w405:string[])
        n161 = Empty String/Path?(string/path="Additional Notes?") -> (empty?=w399:bool)
        n162 = Unbundle By Name(w410) -> ("Log.string"=w408:string)
        n163 = for {
          tunnel: w405 -> [w422] mode=indexing
          tunnel: [w421] -> w404 mode=indexing
          n164 = Concatenate Strings("  - " ("format string"), w422) -> (w421:string)
        }
        n165 = call <userlib>:"1D Array to String__ogtk.vi"("delimiter (Tab)"="\n", "Array of Strings"=w404) -> ("delimited string"=w402:string)  [unwired: 9 in]
        n166 = case shown="True" w399 {
          tunnel: w408 -> [w417 w420]
          tunnel: [w416 w420] -> w407
          tunnel: w406 -> [w415 w419]
          tunnel: w402 -> [w414 _]
          tunnel: [w413 w419] -> w401
          frame False {
            n167 = Format Into String(format string="\n- Notes:\n%s", initial string=w417, error in=w415, w414) -> (resulting string=w416:string, error out=w413:errorcluster)
          }
          frame True {
          }
        }
        n168 = Bundle By Name(cluster=w410, "Log.string"=w407) -> (w409:T3)
        n169 = call <vilib>:"Add State(s) to Queue__JKI_lib_State_Machine.vi"("State(s) in (\"\")"=w412) -> ("States Out"=w411:string)  [unwired: 14 in]
      }
      frame "Log: Add Files" {
        # "Template Separator\n(You can make a copy of, or modify, this frame)"
        n170 = Unbundle By Name(w445) -> ("Log.string"=w442:string, "Converted"=w438:path[], "Failed Conversions"=w437:path[], "Original"=w436:path[])
        n171 = call-poly <userlib>:"Strip Path__ogtk.vi"("path"=w436) -> ("name"=w433:string[])  [unwired: 1 out]
        n172 = call-poly <userlib>:"Strip Path__ogtk.vi"("path"=w437) -> ("name"=w427:string[])  [unwired: 1 out]
        n173 = call-poly <userlib>:"Strip Path__ogtk.vi"("path"=w438) -> ("name"=w428:string[])  [unwired: 1 out]
        n174 = for {
          tunnel: w428 -> [w449] mode=indexing
          tunnel: [w448] -> w430 mode=indexing
          n175 = Concatenate Strings("  - " ("format string"), w449) -> (w448:string)
        }
        n176 = for {
          tunnel: w427 -> [w452] mode=indexing
          tunnel: [w451] -> w431 mode=indexing
          n177 = Concatenate Strings("  - " ("format string"), w452) -> (w451:string)
        }
        n178 = for {
          tunnel: w433 -> [w455] mode=indexing
          tunnel: [w454] -> w435 mode=indexing
          n179 = Concatenate Strings("  - " ("format string"), w455) -> (w454:string)
        }
        n180 = call <userlib>:"1D Array to String__ogtk.vi"("delimiter (Tab)"="\n", "Array of Strings"=w430) -> ("delimited string"=w426:string)  [unwired: 9 in]
        n181 = call <userlib>:"1D Array to String__ogtk.vi"("delimiter (Tab)"="\n", "Array of Strings"=w431) -> ("delimited string"=w425:string)  [unwired: 9 in]
        n182 = call <userlib>:"1D Array to String__ogtk.vi"("delimiter (Tab)"="\n", "Array of Strings"=w435) -> ("delimited string"=w424:string)  [unwired: 9 in]
        n183 = Format Into String(format string="\n\nConverted File:\n%s\n\nFailed Conversions:\n%s\n\nOriginal Files:\n%s", initial string=w442, error in=w441, w426, w425, w424) -> (resulting string=w439:string, error out=w440:errorcluster)
        n184 = Bundle By Name(cluster=w445, "Log.string"=w439) -> (w444:T3)
        n185 = call <vilib>:"Add State(s) to Queue__JKI_lib_State_Machine.vi"("State(s) in (\"\")"=w447) -> ("States Out"=w446:string)  [unwired: 14 in]
      }
      frame "Log: Write File" {
        # "G:\\My Drive\\ansom\\data\\MNK\\SAMPLE\\"
        # "Experiment Folder--Conversion-Log--DATE.txt"
        # "Experiment"
        # "File"
        # "Your code here.\n(You can make a copy of, or modify, this frame)"
        n186 = Unbundle By Name(w471) -> ("Original"=w466:path[], "Log.End Time"=w460:string, "Log.string"=w457:string)
        "resulting string" <- w457
        n187 = Index Array(array=w466) -> (element=w465:path)  [unwired: 1 in]
        n188 = Strip Path(path=w465) -> (stripped path=w464:path)  [unwired: 1 out]
        n189 = Strip Path(path=w464) -> (stripped path=w468:path, name=w459:string)
        n190 = Format Into String(format string="--Conversion--%s.log" ("name or relative path"), error in=w462, w460) -> (resulting string=w469:string, error out=w461:errorcluster)  [unwired: 1 in]
        n191 = Concatenate Strings(w459, w469) -> (w470:string)
        n192 = Build Path(base path=w468, name or relative path=w470) -> (appended path=w458:path)
        "Log File Path" <- w458
        n193 = Write to Text File(file (use dialog)=w458, text=w457, error in=w461) -> (error out=w467:errorcluster)  [unwired: 1 in, 2 out]
        n194 = call <vilib>:"Add State(s) to Queue__JKI_lib_State_Machine.vi"("State(s) in (\"\")"=w473) -> ("States Out"=w472:string)  [unwired: 14 in]
      }
    }
  }
  "error out" <- w4
  n195 = Unbundle By Name(w2) -> ("Conversion.lvclass"=→"Conversion.lvclass out":refnum<class "Conversion.lvclass">)
